vi "Overly Rectange.vi"(8 "error out 2":errorcluster caption="error out", 10 "face_list":T1[](array[typedef]), 11 "Image In":T2) -> (0 "error out":errorcluster, 3 "Image Out":T2)   [LabVIEW 2017]
uses:
  <vilib>/vision/Image Controls.llb/IMAQ Image.ctl
  controls/face_list.ctl
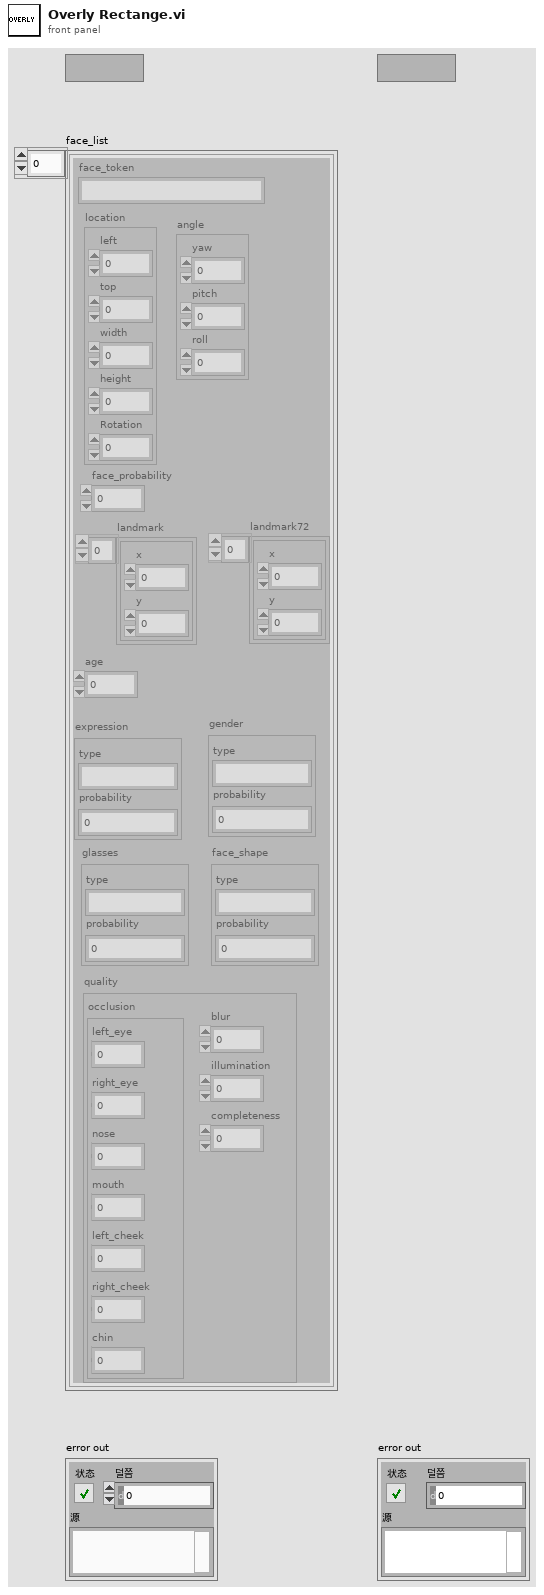
[diagram p1: front panel]
types:
  T1 = typedef "face_list.ctl" = cluster{"location":cluster{"left":i32, "top":i32, "width":i32, "height":i32, "Rotation":i32}, "face_probability":dbl, "age":dbl, "landmark":cluster{"x":u32, "y":u32}[], "landmark72":cluster{"x":u32, "y":u32}[], "angle":cluster{"yaw":dbl, "pitch":dbl, "roll":dbl}, "face_token":string, "face_shape":cluster{"type":string, "probability":dbl}, "glasses":cluster{"type":string, "probability":dbl}, "expression":cluster{"type":string, "probability":dbl}, "gender":cluster{"type":string, "probability":dbl}, "quality":cluster{"illumination":i32, "completeness":i32, "blur":i32, "occlusion":cluster{"left_eye":dbl, "right_eye":dbl, "nose":dbl, "mouth":dbl, "left_cheek":dbl, "right_cheek":dbl, "chin":dbl}}}
  T2 = typedef "IMAQ Image.ctl" = refnum<image>
  T3 = cluster{"left":i32, "top":i32, "width":i32, "height":i32, "Rotation":i32}
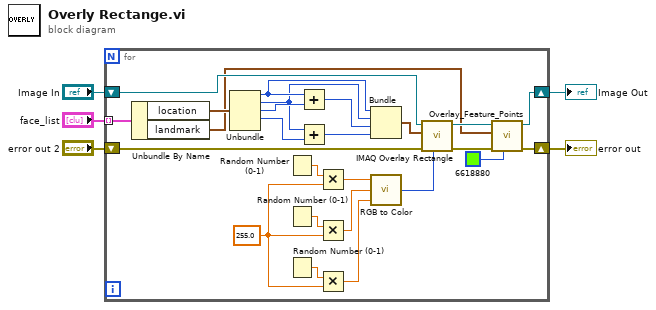
[diagram p0: block diagram]
diagram:
  n1 = for {
    tunnel: "face_list" -> [w22] mode=indexing
    shift-right: [w17] -> w3
    shift-left: "Image In" -> [w30]
    shift-right: [w14] -> w4
    shift-left: "error out 2" -> [w16]
    w6 = 255.0 ("y")
    n2 = Unbundle By Name(w22) -> ("location"=w21:T3, "landmark"=w18:cluster{"x":u32, "y":u32}[])
    n3 = Unbundle(w21) -> ("left"=w27:i32, "top"=w26:i32, "width"=w29:i32, "height"=w28:i32)  [unwired: 1 out]
    n4 = Random Number (0-1)() -> (number: 0 to 1=w13:dbl)
    n5 = Random Number (0-1)() -> (number: 0 to 1=w12:dbl)
    n6 = Random Number (0-1)() -> (number: 0 to 1=w11:dbl)
    n7 = Add(x=w27, y=w29) -> (x+y=w25:i32)
    n8 = Add(x=w26, y=w28) -> (x+y=w24:i32)
    n9 = Multiply(x=w13, y=w6) -> (x*y=w10:dbl)
    n10 = Multiply(x=w12, y=w6) -> (x*y=w9:dbl)
    n11 = Multiply(x=w11, y=w6) -> (x*y=w8:dbl)
    n12 = Bundle("left"=w27, "top"=w26, w25, w24) -> (w23:cluster{"left":i32, "top":i32, i32, i32})  [unwired: 1 in]
    n13 = call <vilib>:"RGB to Color.vi"("B"=w8, "G"=w9, "R"=w10) -> ("Color"=w7:u32)
    n14 = call "IMAQ Overlay Rectangle"("Color"=w7, "error in (no error)"=w16, "Rectangle"=w23, "Image"=w30) -> ("error out"=w15:errorcluster, "Image Out"=w19:T2)  [unwired: 6 in]
    n15 = call "Overlay_Feature_Points.vi"("Color"=u32 6618880, "error in"=w15, "Feature Points"=w18, "Image"=w19) -> ("error out"=w14:errorcluster, "Image Out"=w17:T2)  [unwired: 6 in]
  }
  "Image Out" <- w3
  "error out" <- w4
